vi "action.vi"(0 "HGF_FGV_Select":refnum<class "HGF_FGV_Selection.lvclass">, 2 "Objects":refnum<class>[](array[class]), 5 "error in (no error)":errorcluster) -> (14 "dup HGF_FGV_Select":refnum<class "HGF_FGV_Selection.lvclass">, 16 "dup Objects":refnum<class>[](array[class]), 19 "error out":errorcluster)   [LabVIEW 2012, in "HGF_FGV.lvlib" / "HGF_FGV_Selection.lvclass"]
doc: "Return copy of selected objects from object array."
uses:
  HGF_FGV_Selection.lvclass
  HGF_FGV_Selection.lvclass/HGF_FGV_Selection.ctl
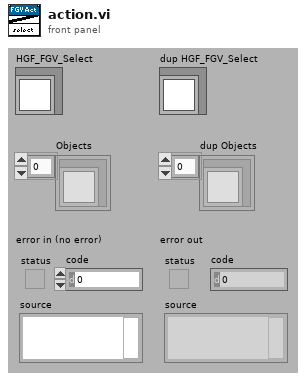
[diagram p1: front panel]
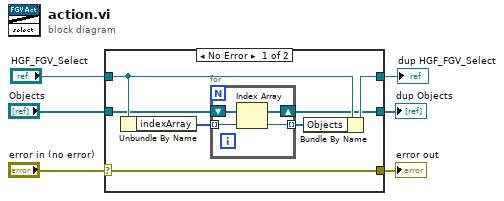
[diagram p0: block diagram]
diagram:
  n1 = case shown="No Error" "error in (no error)" {
    selector: "error in (no error)" -> [w13 w19]
    tunnel: [w13 w19] -> w5
    tunnel: [w12 w18] -> w3
    tunnel: "HGF_FGV_Select" -> [w11 w18]
    tunnel: [w9 w17] -> w2
    tunnel: "Objects" -> [w10 w17]
    frame No Error {
      n2 = Unbundle By Name(w11) -> ("indexArray"=w8:u32[])
      n3 = for {
        shift-right: [w16] -> w9
        shift-left: w10 -> [w16]
        tunnel: w8 -> [w15] mode=indexing
        tunnel: [w14] -> w7 mode=indexing
        n4 = Index Array(array=w16, index=w15) -> (element=w14:refnum<class>)
      }
      n5 = Bundle By Name(cluster=w11, "Objects"=w7) -> (w12:refnum<class "HGF_FGV_Selection.lvclass">)
    }
    frame Error {
    }
  }
  "error out" <- w5
  "dup HGF_FGV_Select" <- w3
  "dup Objects" <- w2
